vi "Celsius to Fahrenheit Converter.vi"() -> ()   [LabVIEW 2013]
panel:
  in  "Loop Seconds Delay":i32=2000
  out "?":string
  out "Celsius":dbl
  out "Fahrenheit":dbl
  out "?":sgl(slide) scale=0.0..250.0
  in  "?":sgl(slide) scale=-100.0..100.0 scale format="%#_3g"
  in  "?":bool
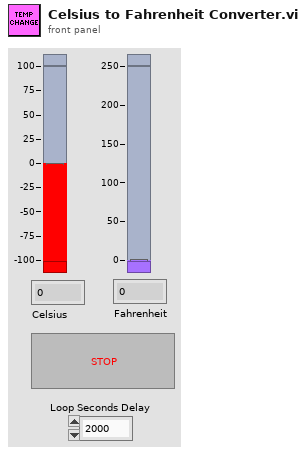
[diagram p1: front panel]
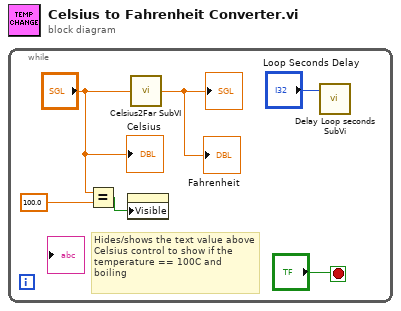
[diagram p0: block diagram]
diagram:
  n1 = while {
    stop <- "?" stop-if-true
    # "Hides/shows the text value above Celsius control to show if the temperature == 100C and boiling"
    n2 = Equal?(x="?", y=100.0) -> (x = y?=w1:bool)
    n3 = property class="Str"("Visible"=w1) -> ()  [unwired: 2 in, 2 out]
    n4 = call "Celsius2Far SubVI.vi"("Celsius in"="?") -> ("Fahrenheit Out"=→"?" →"Fahrenheit":dbl)
    n5 = call "Delay Loop seconds SubVi.vi"("Loop Seconds Delay"="Loop Seconds Delay") -> ()  [unwired: 1 in]
    "Celsius" <- "?"
  }
